vi "Configure Marker Search.vi"(7 "Marker Search":T1(ring), 8 "error in (no error)":errorcluster, 9 "Target Value":dbl, 10 "Marker Number":u8=1, 11 "VNA-Keysight PNA in":refnum<class "VNA-Keysight PNA.lvclass">) -> (0 "error out":errorcluster, 3 "VNA-Keysight PNA out":refnum<class "VNA-Keysight PNA.lvclass">)   [LabVIEW 2020, in "VNA-Keysight PNA.lvclass"]
doc: "Configures and excecutes a marker search.\nThe marker is on the active trace."
uses:
  VNA-Keysight PNA.lvclass
  C:/Sandbox/RF Bench/Source Code/WiSpry Test Framework/Instruments/Instrument.lvclass
  Instrument.lvclass/Instrument.ctl
  Instrument.lvclass
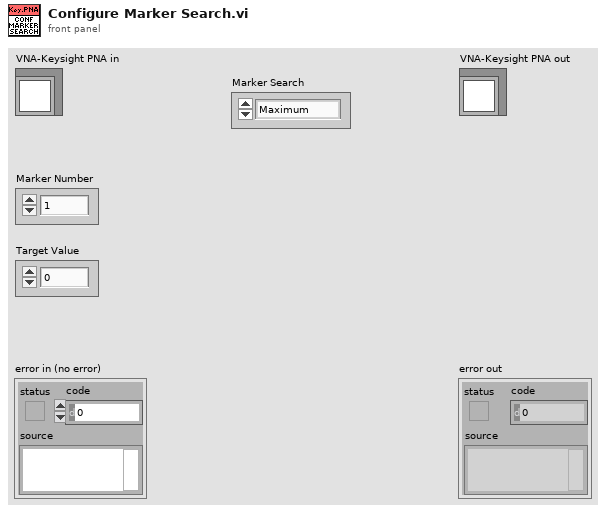
[diagram p1: front panel]
types:
  T1 = enum16{"Maximum", "Minimum", "Right Peak", "Left Peak", "Negative Peak", "Taget Value", "Left Taget Value", "Rigth Target Value"}
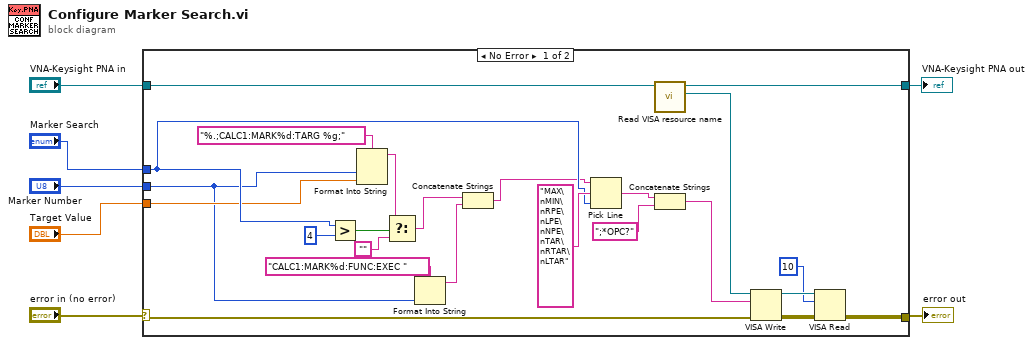
[diagram p0: block diagram]
diagram:
  n1 = case shown="No Error" "error in (no error)" {
    selector: "error in (no error)" -> [w15 w33]
    tunnel: "VNA-Keysight PNA in" -> [w18 w32]
    tunnel: "Marker Search" -> [w30 _]
    tunnel: "Marker Number" -> [w19 _]
    tunnel: "Target Value" -> [w23 _]
    tunnel: [w12 w32] -> w7
    tunnel: [w9 w33] -> w6
    frame No Error {
      n2 = Greater?(x=w30, y=4) -> (0:w29:bool)
      n3 = Format Into String(format string="%.;CALC1:MARK%d:TARG %g;", w19, w23) -> (resulting string=w26:string)  [unwired: 2 in, 1 out]
      n4 = Select(t=w26, s=w29, f="") -> (s? t:f=w25:string)
      n5 = Format Into String(format string="CALC1:MARK%d:FUNC:EXEC ", w19) -> (resulting string=w21:string)  [unwired: 2 in, 1 out]
      n6 = Concatenate Strings(w25, w21) -> (w20:string)
      n7 = Pick Line(string ("")=w20, multi-line string="MAX\nMIN\nRPE\nLPE\nNPE\nTAR\nRTAR\nLTAR", line index=w30) -> (output string=w17:string)
      n8 = call "Read VISA resource name.vi"("Instrument in"=w18) -> ("VISA resource name"=w13:refnum<visa-resource-name>, "Instrument out"=w12:refnum<class "VNA-Keysight PNA.lvclass">)  [unwired: 9 in]
      n9 = Concatenate Strings(w17, ";*OPC?" ("string")) -> (w14:string)
      n10 = VISA Write(VISA resource name=w13, write buffer=w14, error in (no error)=w15) -> (VISA resource name out=w10:refnum<visa-resource-name>, error out=w11:errorcluster)  [unwired: 1 out]
      n11 = VISA Read(VISA resource name=w10, byte count=u32 10, error in (no error)=w11) -> (error out=w9:errorcluster)  [unwired: 3 out]
    }
    frame Error {
    }
  }
  "error out" <- w6
  "VNA-Keysight PNA out" <- w7
